vi "FindToolingPin(SubVI).vi"(0 "Calibrated Image Array":T1[](array[typedef])=["image_000_-618_132_23", "image_001_-618_132_23", "image_002_-618_132_23", "image_006_-338_132_23", "image_007_-338_132_23", "image_008_-338_132_23", "image_012_-44_132_23", "image_013_-44_132_23", "image_014_-44_132_23", "image_018_250_132_23", "image_019_250_132_23", "image_020_250_132_23", "image_003_-606_132_23", "image_004_-606_132_23", "image_005_-606_132_23", "image_009_-326_132_23", "image_010_-326_132_23", "image_011_-326_132_23", "image_015_-32_132_23", "image_016_-32_132_23", "image_017_-32_132_23", "image_021_262_132_23", "image_022_262_132_23", "image_023_262_132_23"], 12 "Templates path":path=path "C:/Users/Aerotech/Documents/BNL_ThermomechanicalStave/0_Calibration") -> (4 "Analyzed Image Array":T1[](array[typedef])=["image_000_-618_132_23", "image_003_-606_132_23", "image_001_-618_132_23", "image_004_-606_132_23", "image_002_-618_132_23", "image_005_-606_132_23", "image_006_-338_132_23", "image_009_-326_132_23", "image_007_-338_132_23", "image_010_-326_132_23", "image_008_-338_132_23", "image_011_-326_132_23", "image_012_-44_132_23", "image_015_-32_132_23", "image_013_-44_132_23", "image_016_-32_132_23", "image_014_-44_132_23", "image_017_-32_132_23", "image_018_250_132_23", "image_021_262_132_23", "image_019_250_132_23", "image_022_262_132_23", "image_020_250_132_23", "image_023_262_132_23"], 8 "Center positions":sgl[][][](array[numeric])=[[[859.75714, 1232.3508, 0.0, 0.0], [0.0, 0.0, 0.0, 0.0]], [[2555.3462, 1299.2568, 0.0, 0.0], [0.0, 0.0, 0.0, 0.0]], [[860.05646, 1232.4283, 0.0, 0.0], [0.0, 0.0, 0.0, 0.0]], [[2558.0, 1310.0, 0.0, 0.0], [0.0, 0.0, 0.0, 0.0]], [[859.81067, 1232.0848, 0.0, 0.0], [0.0, 0.0, 0.0, 0.0]], [[2557.2878, 1299.1604, 0.0, 0.0], [0.0, 0.0, 0.0, 0.0]], [[2327.4531, 2340.4797, 0.0, 0.0], [0.0, 0.0, 0.0, 0.0]], [[1289.3495, 1558.2103, 0.0, 0.0], [0.0, 0.0, 0.0, 0.0]], [[2325.6594, 2341.8496, 0.0, 0.0], [0.0, 0.0, 0.0, 0.0]], [[1286.013, 1558.137, 0.0, 0.0], [0.0, 0.0, 0.0, 0.0]], [[2325.9219, 2341.1997, 0.0, 0.0], [0.0, 0.0, 0.0, 0.0]], [[1289.3192, 1556.233, 0.0, 0.0], [0.0, 0.0, 0.0, 0.0]], [[2378.9963, 2229.6907, 0.0, 0.0], [0.0, 0.0, 0.0, 0.0]], [[1337.5789, 1392.2604, 0.0, 0.0], [0.0, 0.0, 0.0, 0.0]], [[2378.047, 2231.8325, 0.0, 0.0], [0.0, 0.0, 0.0, 0.0]], [[1338.4786, 1392.1888, 0.0, 0.0], [0.0, 0.0, 0.0, 0.0]], [[2379.9888, 2229.9487, 0.0, 0.0], [0.0, 0.0, 0.0, 0.0]], [[1337.3435, 1391.3676, 0.0, 0.0], [0.0, 0.0, 0.0, 0.0]], [[2448.3909, 2123.705, 0.0, 0.0], [0.0, 0.0, 0.0, 0.0]], [[1426.7609, 1386.5051, 0.0, 0.0], [0.0, 0.0, 0.0, 0.0]], [[2447.05, 2123.6472, 0.0, 0.0], [0.0, 0.0, 0.0, 0.0]], [[1428.7585, 1384.3727, 0.0, 0.0], [0.0, 0.0, 0.0, 0.0]], [[2447.701, 2123.5325, 0.0, 0.0], [0.0, 0.0, 0.0, 0.0]], [[1428.5219, 1383.686, 0.0, 0.0], [0.0, 0.0, 0.0, 0.0]]])   [LabVIEW 2016]
uses:
  <vilib>/vision/Image Controls.llb/IMAQ Image.ctl
panel:
  in  "Templates path 2":path=path "C:/Users/Aerotech/Documents/BNL_ThermomechanicalStave/0_Calibration"
  out "Template Image 2":T1
  out "Matches (pixel) Bottom":T2(array[cluster])
  out "Matches (pixel)":T2(array[cluster])
  in  "Search Rect":T3={"Left"=0, "Top"=0, "Right"=2147483647, "Bottom"=2147483647, "Rotation"=0.0} {"Rotation" format="%.2f"; "Left" scale=0.0..1024.0; "Right" scale=0.0..1024.0}
  in  "Pattern Match Settings":T4={"Algorithm"=2, "Number of Matches Requested"=1, "Minimum Match Score"=600.0, "SubPixel Accuracy"=TRUE, "Rotation Angle Ranges"=[{"Start"=0.0, "End"=360.0}], "Show Search Area"=FALSE, "Show Result"=TRUE} {"Rotation Angle Ranges"."End" format="%.1f"; "Rotation Angle Ranges"."Start" format="%.1f"; "Minimum Match Score" min=0 max=1000 format="%.2f"; "Number of Matches Requested" min=1; "Algorithm" items=["All", "Low Discrepancy Sampling", "Grayscale Value Pyramid", "Gradients Pyramid"]}
  out "Template Image":T1
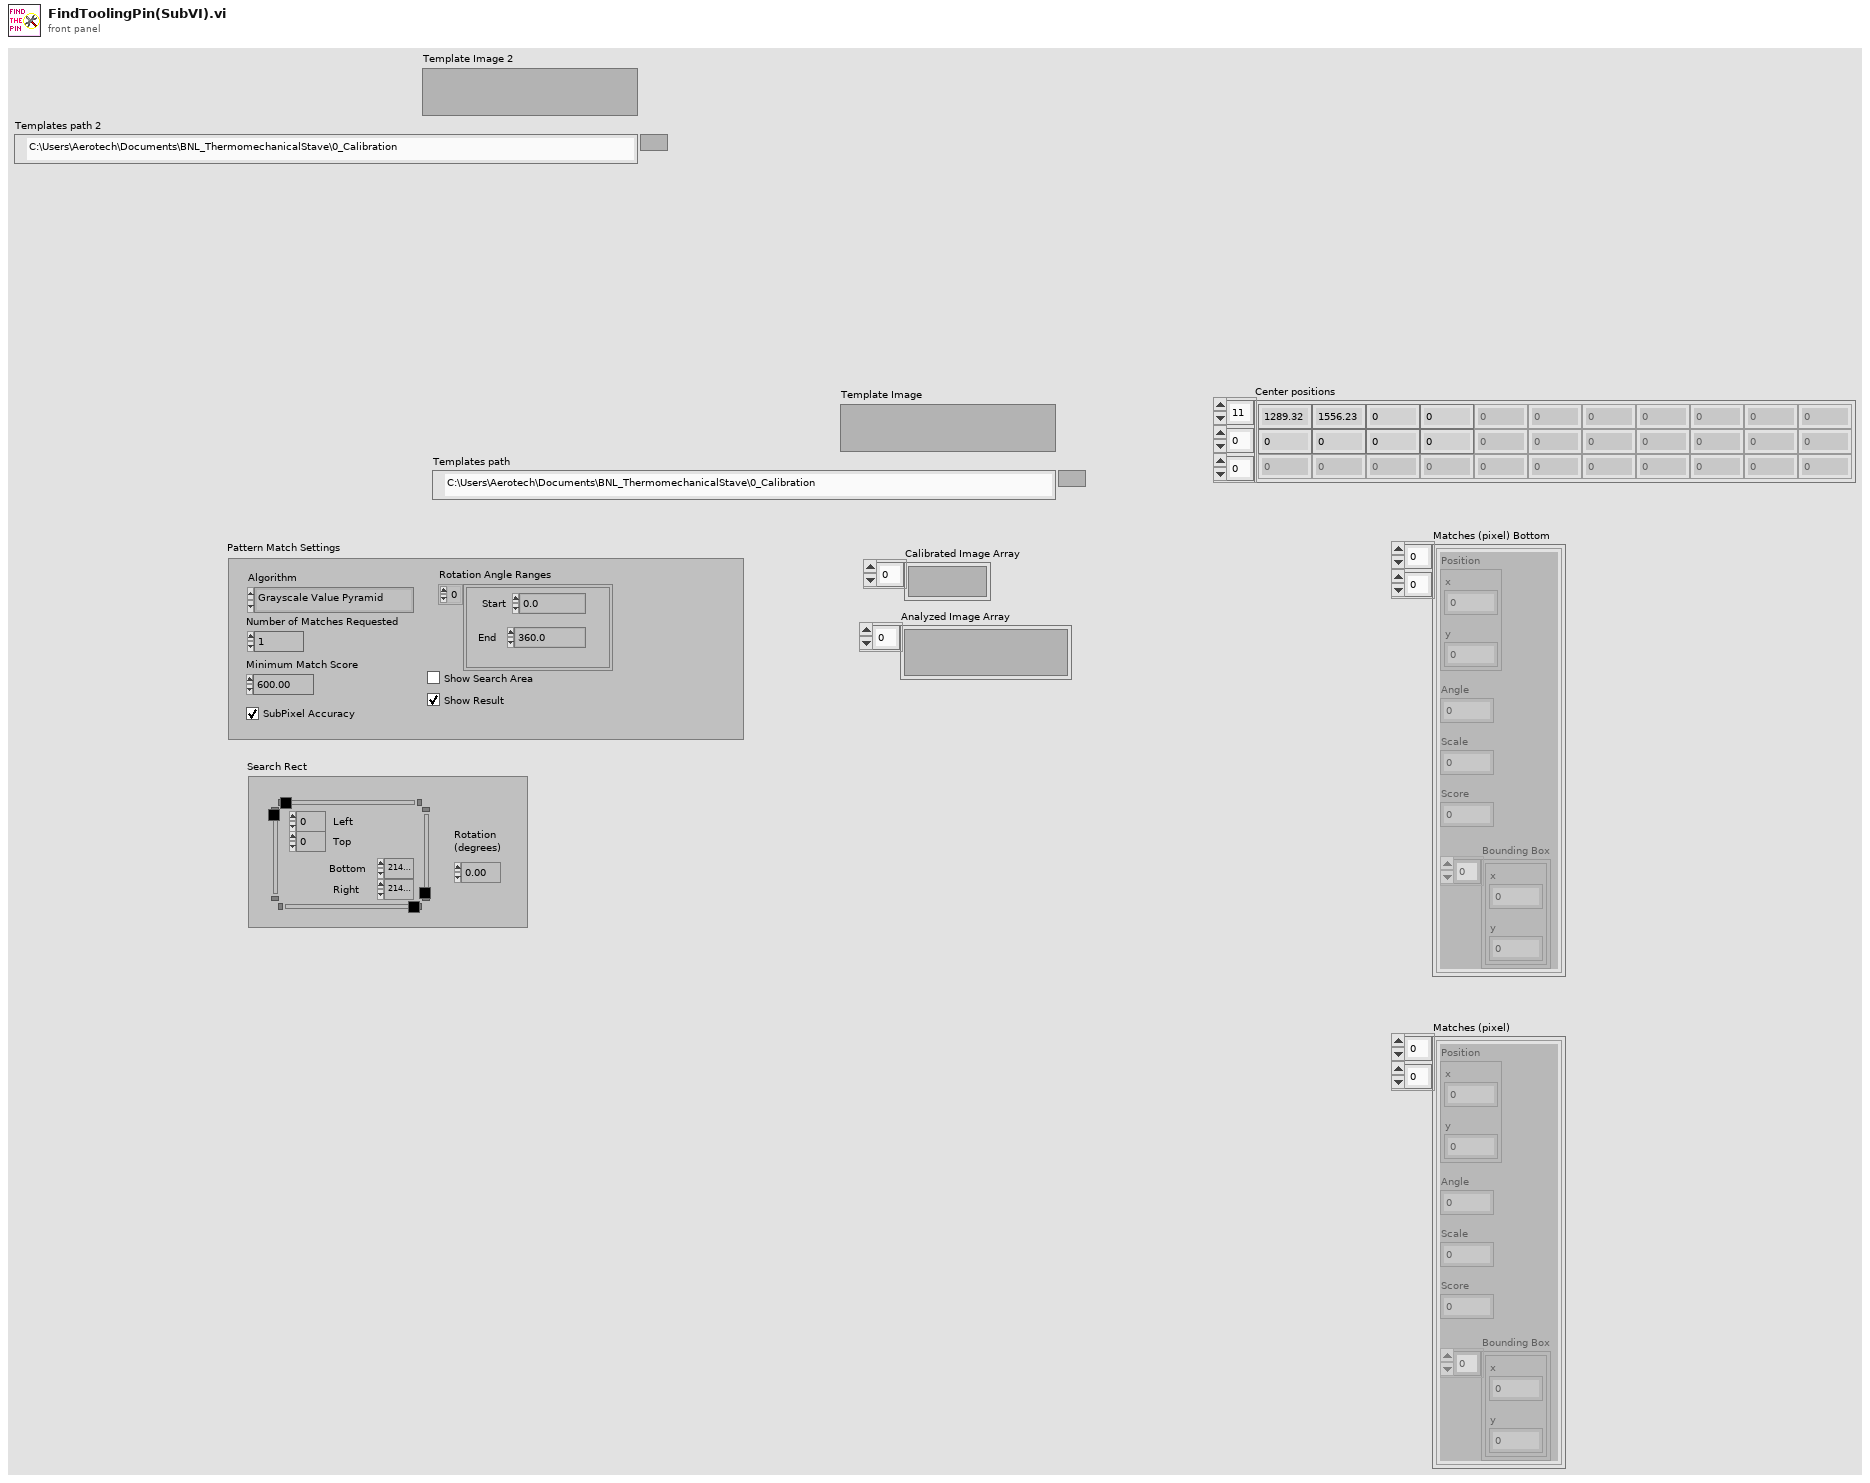
[diagram p1: front panel]
types:
  T1 = typedef "IMAQ Image.ctl" = refnum<image>
  T2 = cluster{"Position":cluster{"x":sgl, "y":sgl}, "Angle":sgl, "Scale":sgl, "Score":sgl, "Bounding Box":cluster{"x":sgl, "y":sgl}[]}[][]
  T3 = typedef "IMAQ Rectangle" = cluster{"Left":i32, "Top":i32, "Right":i32, "Bottom":i32, "Rotation":dbl}
  T4 = cluster{"Algorithm":i32, "Number of Matches Requested":i32, "Minimum Match Score":sgl, "SubPixel Accuracy":bool, "Rotation Angle Ranges":cluster{"Start":sgl, "End":sgl}[], "Show Search Area":bool, "Show Result":bool}
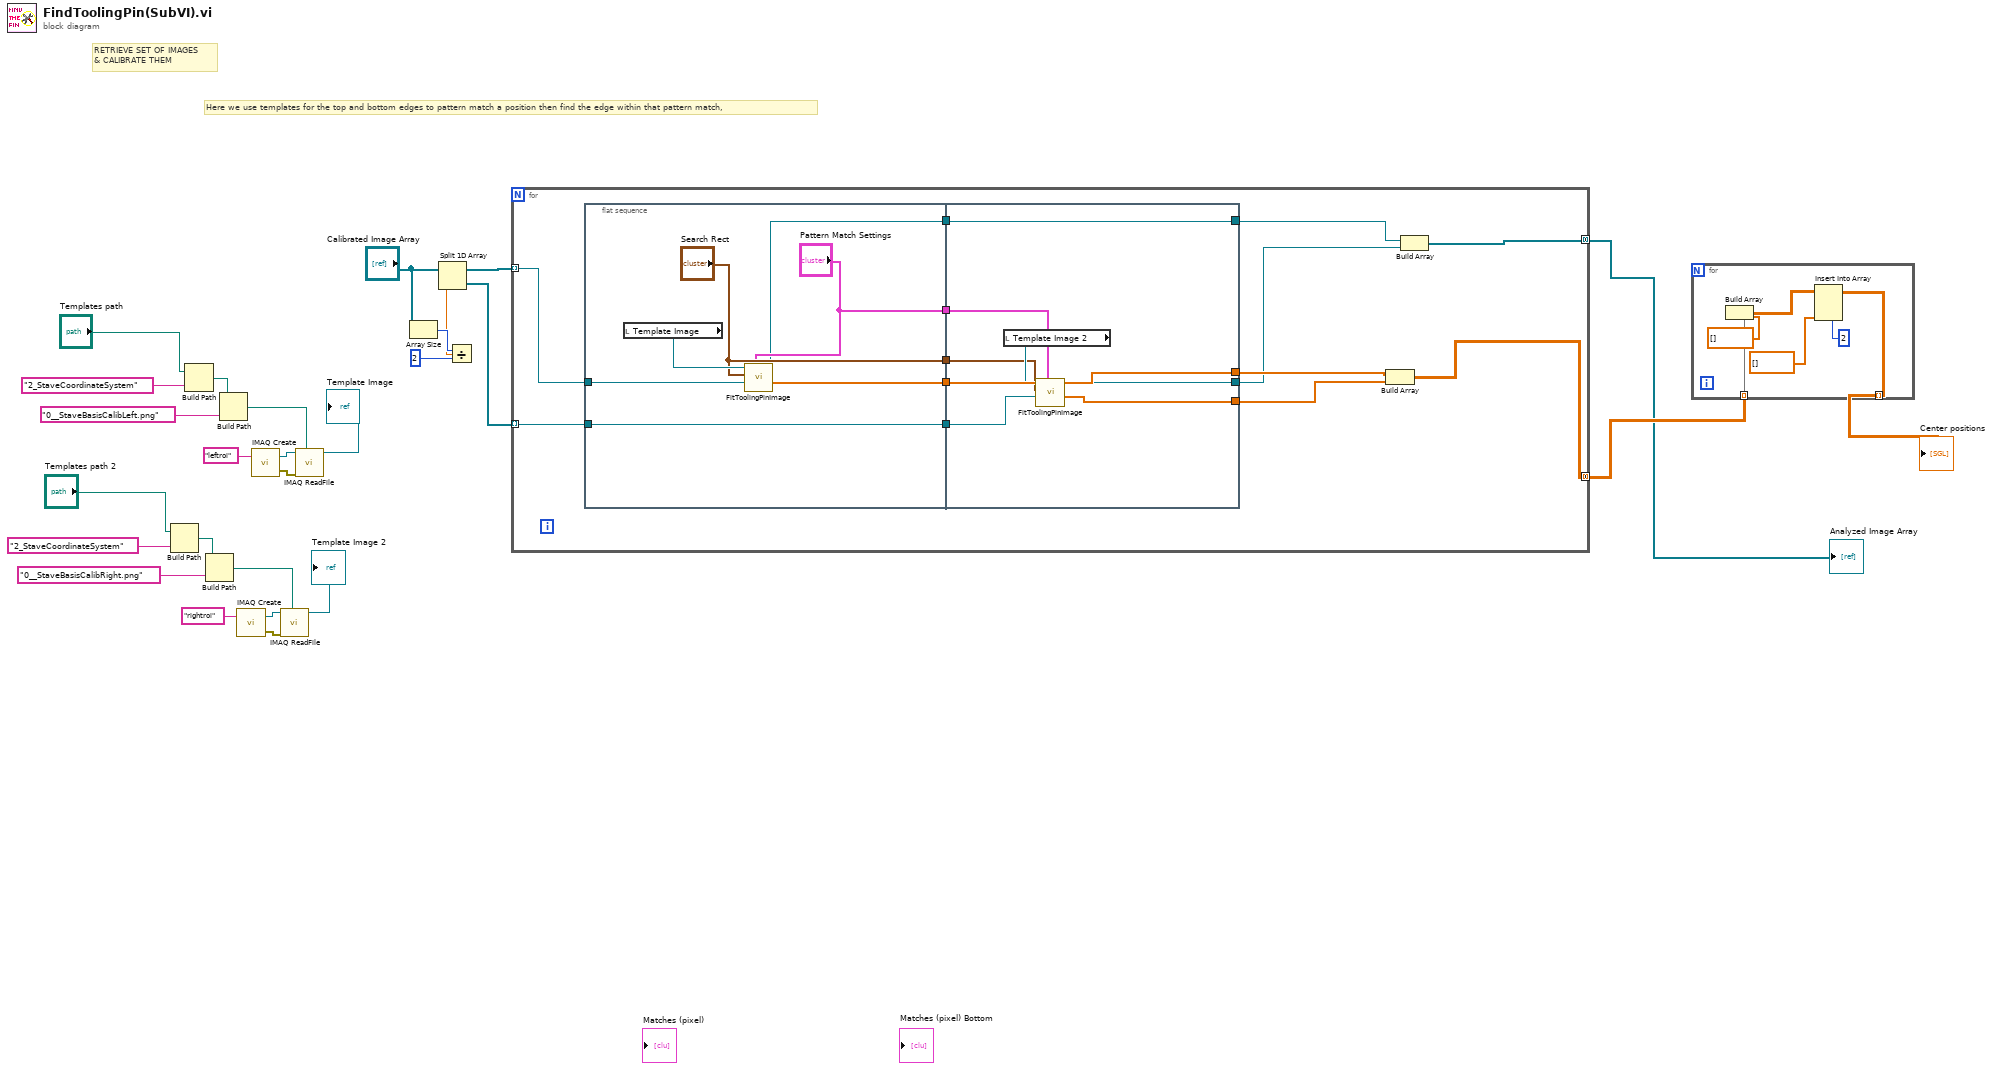
[diagram p0: block diagram]
diagram:
  # "RETRIEVE SET OF IMAGES\n& CALIBRATE THEM"
  # "Here we use templates for the top and bottom edges to pattern match a position then find the edge within that pattern match,"
  n1 = Build Path(base path="Templates path 2", name or relative path="2_StaveCoordinateSystem") -> (appended path=w3:path)
  n2 = Build Path(base path="Templates path", name or relative path="2_StaveCoordinateSystem") -> (appended path=w19:path)
  n3 = Build Path(base path=w3, name or relative path="0__StaveBasisCalibRight.png") -> (appended path=w4:path)
  n4 = Build Path(base path=w19, name or relative path="0__StaveBasisCalibLeft.png") -> (appended path=w20:path)
  n5 = call "IMAQ Create"("Image Name"="rightroi") -> ("New Image"=w8:T1, "error out"=w9:errorcluster)  [unwired: 4 in]
  n6 = call "IMAQ Create"("Image Name"="leftroi") -> ("New Image"=w25:T1, "error out"=w26:errorcluster)  [unwired: 4 in]
  n7 = call "IMAQ ReadFile"("File Path"=w4, "error in (no error)"=w9, "Image"=w8) -> ("Image Out"=→"Template Image 2":T1)  [unwired: 4 in, 4 out]
  n8 = call "IMAQ ReadFile"("File Path"=w20, "error in (no error)"=w26, "Image"=w25) -> ("Image Out"=→"Template Image":T1)  [unwired: 4 in, 4 out]
  n9 = Array Size(array="Calibrated Image Array") -> (size(s)=w13:i32)
  n10 = Divide(x=w13, y=2) -> (x/y=w11:dbl)
  n11 = Split 1D Array(array="Calibrated Image Array", index=w11) -> (first subarray=w16:T1[], second subarray=w15:T1[])
  n12 = for {
    tunnel: w16 -> [w40] mode=indexing
    tunnel: [w37] -> w18 mode=concatenating
    tunnel: w15 -> [w28] mode=indexing
    tunnel: [w39] -> w1 mode=concatenating
    n13 = flat-sequence {
      tunnel: w40 -> [w42]
      tunnel: ["Search Rect"] -> w36
      tunnel: ["Pattern Match Settings"] -> w35
      tunnel: [w44] -> w34
      tunnel: [w43] -> w33
      tunnel: [w41] -> w29
      tunnel: w28 -> [w41]
      tunnel: [w54] -> w32
      tunnel: [w55] -> w38
      tunnel: w36 -> [w50]
      tunnel: w35 -> [w49]
      tunnel: w34 -> [w55]
      tunnel: w33 -> [w54]
      tunnel: [w52] -> w31
      tunnel: [w51] -> w30
      tunnel: w29 -> [w48]
      frame #0 {
        n14 = local read "Template Image"() -> (w47:T1)
        n15 = call "FitToolingPinImage.vi"("Pattern Match Settings"="Pattern Match Settings", "Calibrated Image"=w42, "Search Rect"="Search Rect", "Template"=w47) -> ("Corner positions"=w43:sgl[], "Refnum out"=w44:T1)  [unwired: 6 in]
      }
      frame #1 {
        n16 = local read "Template Image 2"() -> (w53:T1)
        n17 = call "FitToolingPinImage.vi"("Pattern Match Settings"=w49, "Calibrated Image"=w48, "Search Rect"=w50, "Template"=w53) -> ("Corner positions"=w52:sgl[], "Refnum out"=w51:T1)  [unwired: 6 in]
      }
    }
    n18 = Build Array(w32, w31) -> (w37:sgl[][])
    n19 = Build Array(w38, w30) -> (w39:T1[])
  }
  "Analyzed Image Array" <- w1
  n20 = for {
    tunnel: w18 -> [w56] mode=indexing
    tunnel: [w57] -> w17 mode=indexing
    n21 = Build Array(w56, dbl[] [] ("element")) -> (w60:dbl[][])
    n22 = Insert Into Array(array=w60, index (col)=2 ("disabled index (col)"), new element=dbl[] [] ("new element/subarray")) -> (w57:dbl[][])  [unwired: 1 in]
  }
  "Center positions" <- w17
